vi "DIO Bit Read.vi"(8 "error in (no error)":errorcluster, 9 "Line":string, 10 "Port":string, 11 "DIO Device":tag) -> (0 "error out":errorcluster, 2 "data":bool)   [LabVIEW 2022 SP3, in "niMIO.lvclass"]
uses:
  niMIO.lvclass
  <vilib>/DAQmx/read.llb/DAQmx Read (Digital Bool 1Line 1Point).vi
  <vilib>/DAQmx/create/channels.llb/DAQmx Create Channel (DI-Digital Input).vi
  <vilib>/DAQmx/miscellaneous.llb/DAQmx Fill In Error Info.vi
  niMIO.lvclass/niMIO.ctl
panel:
  out "niDIO out":refnum<class "niMIO.lvclass">
  in  "niDIO in":refnum<class "niMIO.lvclass">
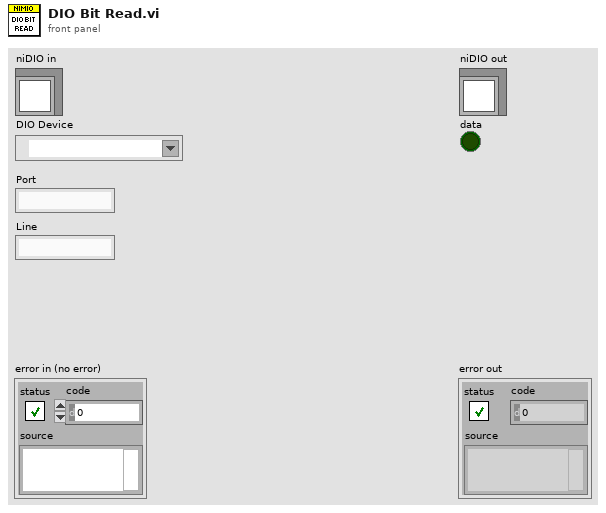
[diagram p1: front panel]
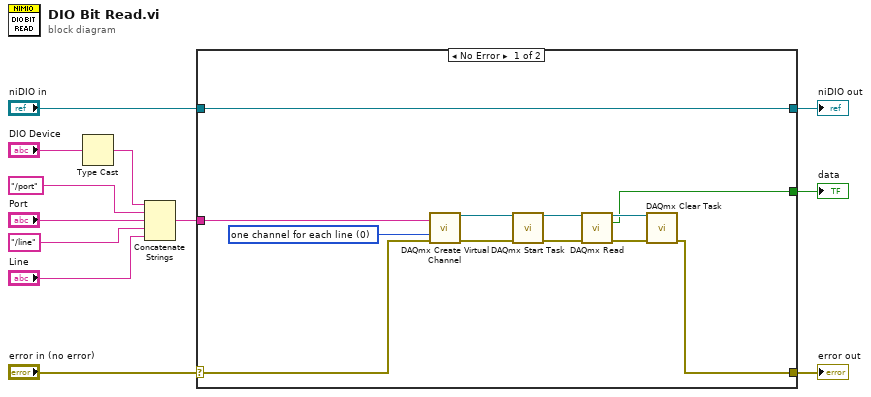
[diagram p0: block diagram]
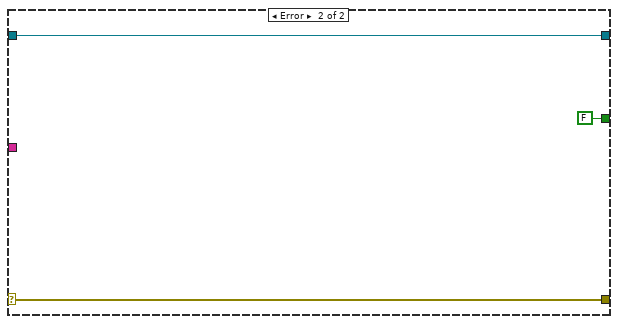
[diagram p2: hidden frame]
diagram:
  n1 = Type Cast(x="DIO Device") -> (*(type *) &x=w3:string)  [unwired: 1 in]
  n2 = Concatenate Strings(w3, "/port", "Port", "/line" ("string"), "Line") -> (w1:string)
  n3 = case shown="No Error" "error in (no error)" {
    selector: "error in (no error)" -> [w15 w27]
    tunnel: [w14 w27] -> w11
    tunnel: [w24 w26] -> w9
    tunnel: "niDIO in" -> [w24 w26]
    tunnel: w1 -> [w16 _]
    tunnel: [w13 FALSE ("data")] -> w8
    frame No Error {
      w21 = 0 items=["one channel for each line", "one channel for all lines"] ("line grouping")
      n4 = call-poly <vilib>:"DAQmx Create Virtual Channel.vi"("lines"=w16, "line grouping"=w21, "error in"=w15) -> ("task out"=w23:refnum<k21>, "error out"=w22:errorcluster)  [unwired: 11 in]
      n5 = call <vilib>:"DAQmx Start Task.vi"("task/channels in"=w23, "error in"=w22) -> ("task out"=w20:refnum<k21>, "error out"=w19:errorcluster)  [unwired: 12 in]
      n6 = call-poly <vilib>:"DAQmx Read.vi"("task/channels in"=w20, "error in"=w19) -> ("task out"=w18:refnum<k21>, "data"=w13:bool, "error out"=w17:errorcluster)  [unwired: 11 in]
      n7 = call <vilib>:"DAQmx Clear Task.vi"("task in"=w18, "error in"=w17) -> ("error out"=w14:errorcluster)  [unwired: 13 in]
    }
    frame Error {
    }
  }
  "error out" <- w11
  "niDIO out" <- w9
  "data" <- w8
